vi "logTestAuto2.vi"(0 "att dB":u8, 3 "comments":string, 4 "TSfile":string="baseline.tim" caption="Path to user TS", 5 "currVolts":dbl min=0.0 max=15.0 step=1.0 format="%_3f", 6 "TM":bool, 7 "Test type":T1(ring), 8 "RC":u8=3 format="%b", 9 "AF1":bool, 10 "Gain":u8=8 format="%b", 11 "Chip numberASPIC":string(combo)="03") -> ()   [LabVIEW 2014]
uses:
  Global 1.vi
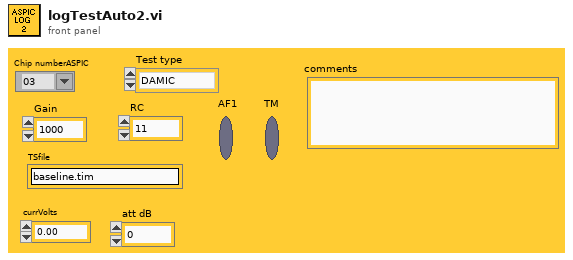
[diagram p1: front panel]
types:
  T1 = enum16{"DAMIC", "NOISE", "GAIN", "LINEAR18", "XTALK", "TEMP", "LINEAR16"}
  T2 = enum16{"open", "replace", "create", "open or create", "replace or create", "replace or create with confirmation"}
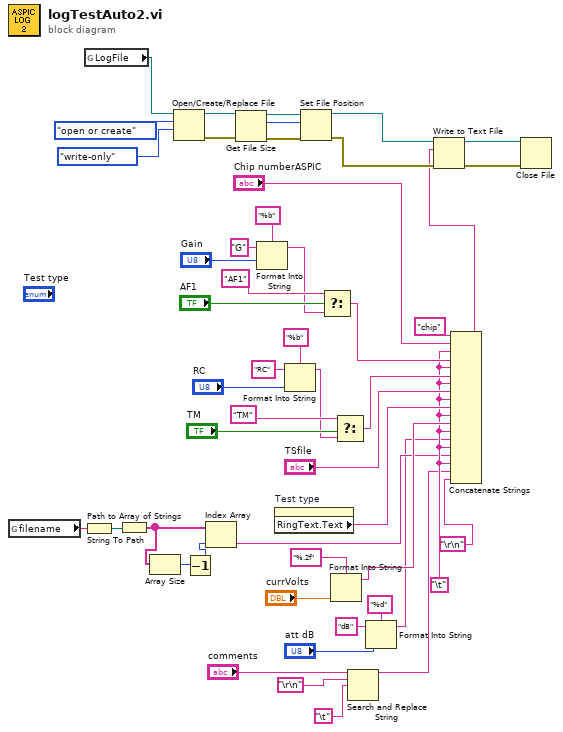
[diagram p0: block diagram]
diagram:
  w7 = "\t"
  n1 = global read "Global 1.vi" "filename"() -> (w50:string)
  n2 = String To Path(string=w50) -> (path=w49:path)
  n3 = global read "Global 1.vi" "LogFile"() -> (w9:path)
  n4 = Path to Array of Strings(0:w49) -> (2:w48:string[])  [unwired: 1 out]
  n5 = Array Size(array=w48) -> (size(s)=w47:i32)
  n6 = Open/Create/Replace File(file path (use dialog)=w9, operation (0:open)=T2."open or create", access (0:read/write)=enum16{"read/write", "read-only", "write-only"}."write-only") -> (refnum out=w43:refnum<file>, error out=w41:errorcluster)  [unwired: 1 in, 3 out]
  n7 = Decrement(x=w47) -> (x-1=w46:i32)
  n8 = Index Array(array=w48, index=w46) -> (element=w2:string)
  n9 = Get File Size(file=w43, error in=w41) -> (refnum out=w42:refnum<file>, size (in bytes)=w39:i64, 0:w40:errorcluster)
  n10 = Format Into String(format string="%b", initial string="G", "Gain") -> (resulting string=w27:string)  [unwired: 1 in, 1 out]
  n11 = property on="Test type" class="Enum (strict)"() -> ("RingText.Text"=w18:string)  [unwired: 2 in, 2 out]
  n12 = Format Into String(format string="%b", initial string="RC", "RC") -> (resulting string=w23:string)  [unwired: 1 in, 1 out]
  n13 = Set File Position(offset (in bytes) (0)=w39, refnum=w42, error in=w40) -> (refnum out=w38:refnum<file>, error out=w31:errorcluster)  [unwired: 1 out]
  n14 = Select(t="AF1", s="AF1", f=w27) -> (s? t:f=w21:string)
  n15 = Format Into String(format string="%.2f", "currVolts") -> (resulting string=w16:string)  [unwired: 2 in, 1 out]
  n16 = Select(t="TM", s="TM", f=w23) -> (s? t:f=w20:string)
  n17 = Search and Replace String(input string="comments", search string="\r\n", replace string="\t") -> (result string=w6:string)  [unwired: 1 in, 7 out]
  n18 = Format Into String(format string="%d", initial string="dB", "att dB") -> (resulting string=w1:string)  [unwired: 1 in, 1 out]
  n19 = Concatenate Strings("chip" ("string"), "Chip numberASPIC", w7, w21, w7, w20, w7, "TSfile", w7, w18, w7, w16, w7, w1, w7, w2, w7, w6, "\r\n") -> (w15:string)
  n20 = Write to Text File(file (use dialog)=w38, text=w15, error in=w31) -> (refnum out=w37:refnum<file>, error out=w30:errorcluster)  [unwired: 2 out]
  n21 = Close File(refnum=w37, error in=w30) -> ()  [unwired: 2 out]
